vi "SetRelativePositionUm.vi"(8 "error in (no error)":errorcluster, 9 "RelativeMoveum":dbl min=0.0 max=200.0, 10 "Stage Label":string, 11 "DemoStepMotor in":refnum<class "DemoStepMotor.lvclass">) -> (0 "error out":errorcluster, 3 "DemoStepMotor out":refnum<class "DemoStepMotor.lvclass">)   [LabVIEW 2020, in "DemoStepMotor.lvlib" / "DemoStepMotor.lvclass"]
uses:
  DemoStepMotor.lvclass
  <vilib>/ActorFramework/Actor/Actor.lvclass
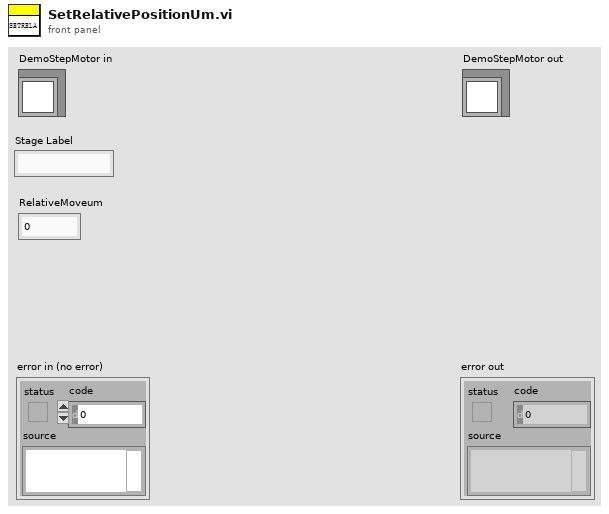
[diagram p1: front panel]
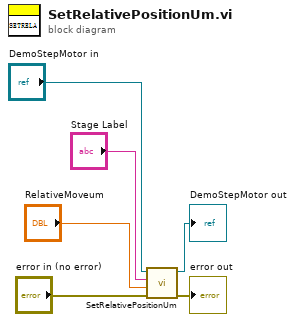
[diagram p0: block diagram]
diagram:
  n1 = call-parent "SetRelativePositionUm.vi"("error in (no error)"="error in (no error)", "RelativeMoveum"="RelativeMoveum", "Stage Label"="Stage Label", "Stage in"="DemoStepMotor in") -> ("error out"=→"error out":errorcluster, "Stage out"=→"DemoStepMotor out":refnum<class "DemoStepMotor.lvclass">)  [unwired: 6 in]
